vi "FGZ.vi"(3 "error in (no error)":errorcluster, 4 "state":T1, 5 "Input":i32) -> (0 "error out":errorcluster, 2 "Output":i32)   [LabVIEW 2024]
uses:
  states.ctl
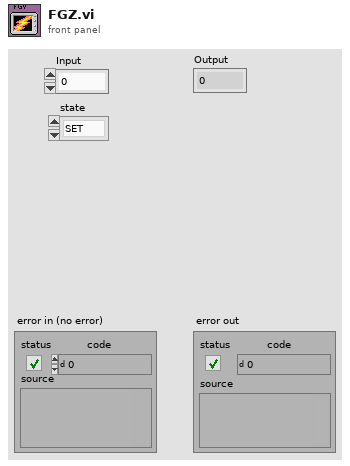
[diagram p1: front panel]
types:
  T1 = typedef "states.ctl" = enum16{"SET", "GET", "INC", "DEC"}
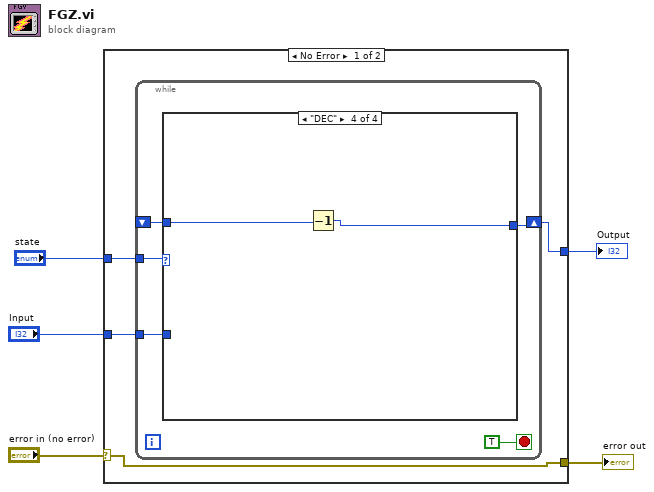
[diagram p0: block diagram]
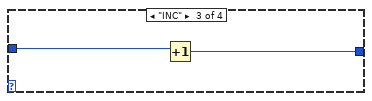
[diagram p4: hidden frame]
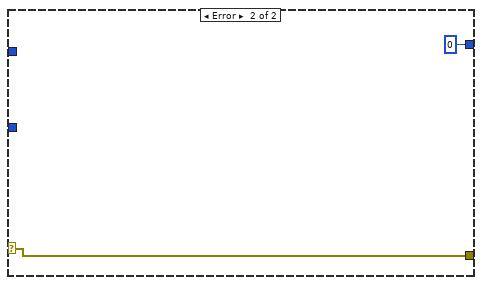
[diagram p5: hidden frame]
diagram:
  n1 = case shown="No Error" "error in (no error)" {
    selector: "error in (no error)" -> [w9 w22]
    tunnel: [w9 w22] -> w4
    tunnel: "state" -> [w8 _]
    tunnel: [w7 0 ("Input")] -> w2
    tunnel: "Input" -> [w6 _]
    frame No Error {
      n2 = while {
        tunnel: w8 -> [w13]
        shift-right: [w11] -> w7
        shift-left: _ -> [w12]
        tunnel: w6 -> [w10]
        stop <- TRUE stop-if-true
        n3 = case shown="\"DEC\"" w13 {
          tunnel: w12 -> [_ w16 w18 w20]
          tunnel: [w15 w16 w17 w19] -> w11
          tunnel: w10 -> [w15 _ _ _]
          frame "SET", Default {
          }
          frame "GET" {
          }
          frame "INC" {
            n4 = Increment(x=w18) -> (x+1=w17:i32)
          }
          frame "DEC" {
            n5 = Decrement(x=w20) -> (x-1=w19:i32)
          }
        }
      }
    }
    frame Error {
    }
  }
  "error out" <- w4
  "Output" <- w2
